vi "Initialize VeriStand Globals.vi"(8 "error in (no error)":errorcluster) -> (0 "error out":errorcluster)   [LabVIEW 2024, in "AIM ARINC 429 Engine.lvlib" / "Custom Device.lvlib"]
uses:
  Custom Device.lvlib
  <vilib>/NI VeriStand/Custom Device API/Data Table Ref.ctl
  <vilib>/NI VeriStand/Custom Device API/Global Data Refs.vi
  <vilib>/NI VeriStand/Custom Device API/Custom Device API.lvlib
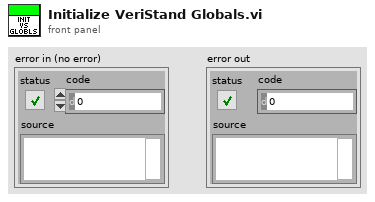
[diagram p1: front panel]
types:
  T1 = typedef "Custom Device API.lvlib/Data Table Ref.ctl" = cluster{"Ptr.Beg":u64, "Ptr.End":u64}
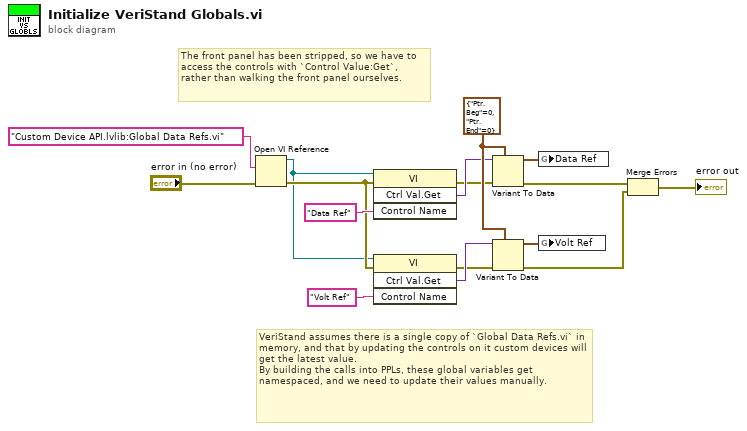
[diagram p0: block diagram]
diagram:
  w13 = T1 {"Ptr.Beg"=0, "Ptr.End"=0} ("Volt Ref")
  # "The front panel has been stripped, so we have to access the controls with `Control Value:Get`, rather than walking the front panel ourselves."
  # "VeriStand assumes there is a single copy of `Global Data Refs.vi` in memory, and that by updating the controls on it custom devices will get the latest value. \nBy building the calls into PPLs, these global variables get namespaced, and we need to update their values manually."
  n1 = Open VI Reference(vi path="Custom Device API.lvlib:Global Data Refs.vi", error in (no error)="error in (no error)") -> (vi reference=w4:refnum<vi>, error out=w6:errorcluster)  [unwired: 4 in]
  n2 = invoke class="VI" method="Ctrl Val.Get"(reference=w4, error in=w6, "Control Name"="Data Ref" ("y")) -> (error out=w7:errorcluster, "Get Control Value Variant"=w8:variant)  [unwired: 1 in, 2 out]
  n3 = invoke class="VI" method="Ctrl Val.Get"(reference=w4, error in=w6, "Control Name"="Volt Ref" ("y")) -> (error out=w2:errorcluster, "Get Control Value Variant"=w3:variant)  [unwired: 1 in, 2 out]
  n4 = Variant To Data(error in=w7, type=w13, Variant=w8) -> (data=w1:T1, error out=w11:errorcluster)
  n5 = Variant To Data(error in=w2, type=w13, Variant=w3) -> (data=w12:T1, error out=w10:errorcluster)
  n6 = global write "Global Data Refs.vi" "Data Ref"(w1) -> ()
  n7 = global write "Global Data Refs.vi" "Volt Ref"(w12) -> ()
  n8 = Merge Errors(w11, w10) -> (→"error out":errorcluster)
